vi "Check for Empty Command Or Response.vi"(7 "Command/Response Refnum in":T1 format="%.0x", 8 "Error In":errorcluster, 11 "Response Format in":string) -> (0 "Error Out":errorcluster, 3 "Response Format out":string)   [LabVIEW 2018, in "Instrument Addon Scripting API.lvlib"]
uses:
  Instrument Addon Scripting API.lvlib
  <vilib>/NI Veristand/Custom Device API/Custom Device Item Ref.ctl
  <vilib>/NI VeriStand/Custom Device API/Custom Device API.lvlib
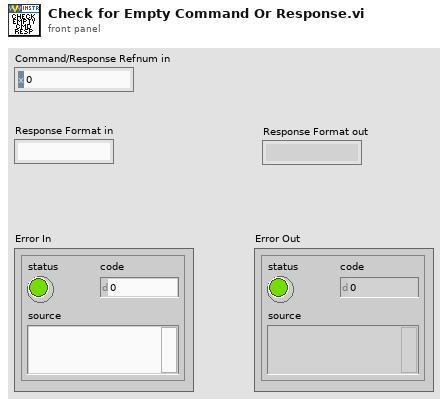
[diagram p1: front panel]
types:
  T1 = typedef "Custom Device API.lvlib/Custom Device Item Ref.ctl" = u64
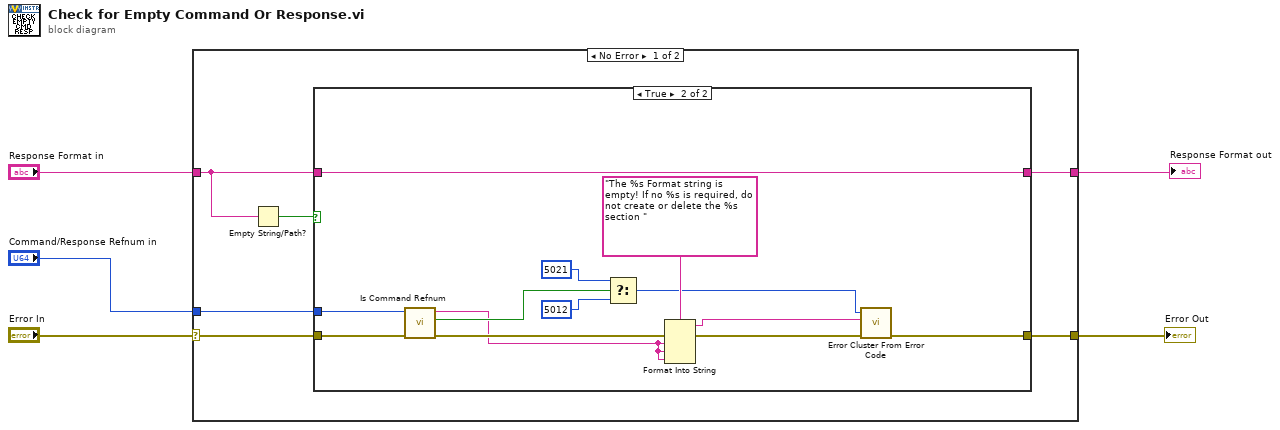
[diagram p0: block diagram]
diagram:
  n1 = case shown="No Error" "Error In" {
    selector: "Error In" -> [w8 w27]
    tunnel: "Response Format in" -> [w10 w28]
    tunnel: [w9 w28] -> w4
    tunnel: [w7 w27] -> w2
    tunnel: "Command/Response Refnum in" -> [w6 _]
    frame No Error {
      n2 = Empty String/Path?(string/path=w10) -> (empty?=w11:bool)
      n3 = case shown="True" w11 {
        tunnel: w10 -> [w13 w26]
        tunnel: [w13 w26] -> w9
        tunnel: w8 -> [w12 w19]
        tunnel: [w12 w25] -> w7
        tunnel: w6 -> [_ w17]
        frame False {
        }
        frame True {
          n4 = call "Is Command Refnum.vi"("error in (no error)"=w19, "Command/Response Refnum in"=w17) -> ("error out"=w23:errorcluster, "Is Command?"=w24:bool, "Command/Response out"=w14:string)  [unwired: 7 in]
          n5 = Select(t=5021 ("error code (0)"), s=w24, f=5012 ("error code (0)")) -> (s? t:f=w16:i32)
          n6 = Format Into String(format string="The %s Format string is empty! If no %s is required, do not create or delete the %s section " ("error message (\"\")"), error in=w23, w14, w14, w14) -> (resulting string=w15:string, error out=w18:errorcluster)  [unwired: 1 in]
          n7 = call <vilib>:"Error Cluster From Error Code.vi"("error in (no error)"=w18, "error message (\"\")"=w15, "error code (0)"=w16) -> ("error out"=w25:errorcluster)  [unwired: 6 in]
        }
      }
    }
    frame Error {
    }
  }
  "Response Format out" <- w4
  "Error Out" <- w2
